vi "Get Exponent of a Number (U32).vi"(9 "Input Valid":bool=TRUE, 10 "Binary Number":u32 format="%.0b") -> (1 "Output Valid":bool, 2 "Exponent":u8, 5 "Binary Number":u32)   [LabVIEW 2011]
uses:
  <vilib>/rvi/FXPMathLib/basic elements/FxpDiscreteDelay/XNode/nifxpmath_DiscreteDelay.xnode
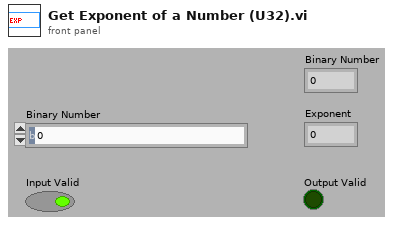
[diagram p1: front panel]
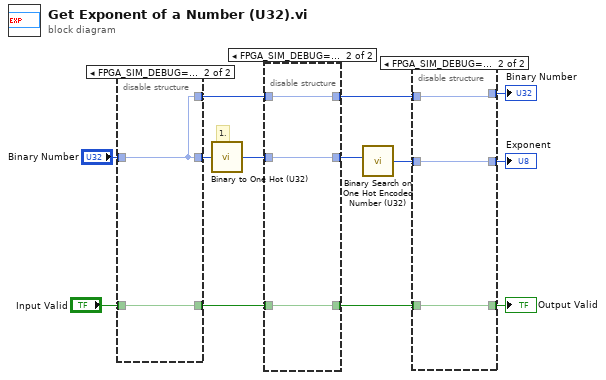
[diagram p0: block diagram]
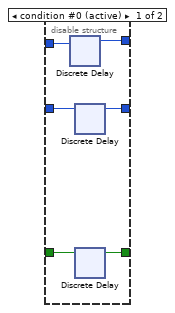
[diagram p2: hidden frame]
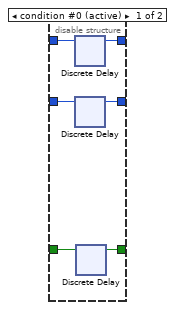
[diagram p3: hidden frame]
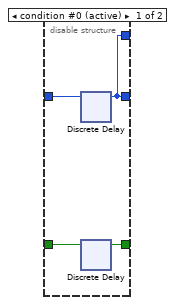
[diagram p4: hidden frame]
diagram:
  # "1."
  n1 = disable-structure shown="FPGA_SIM_DEBUG==TRUE" {
    disable-tunnel: [w14 w18] -> w13
    disable-tunnel: "Input Valid" -> [w17 w19]
    disable-tunnel: [w16 w19] -> w11
    disable-tunnel: "Binary Number" -> [w15 w18]
    disable-tunnel: [w14 w18] -> w3
    frame condition #0 (active) {
      n2 = xnode "Discrete Delay"("D"=w15) -> ("Q"=w14:u32)
      n3 = xnode "Discrete Delay"("D"=w17) -> ("Q"=w16:bool)
    }
    frame condition #1 {
    }
  }
  n4 = call <userlib>:"Binary to One Hot (U32).vi"("Binary Number"=w13) -> ("One Hot Encoded Number"=w9:u32)  [unwired: 14 in]
  n5 = disable-structure shown="FPGA_SIM_DEBUG==TRUE" {
    disable-tunnel: w11 -> [w25 w27]
    disable-tunnel: [w24 w27] -> w10
    disable-tunnel: w9 -> [w23 w28]
    disable-tunnel: [w22 w28] -> w8
    disable-tunnel: w3 -> [w21 w26]
    disable-tunnel: [w20 w26] -> w2
    frame condition #0 (active) {
      n6 = xnode "Discrete Delay"("D"=w21) -> ("Q"=w20:u32)
      n7 = xnode "Discrete Delay"("D"=w23) -> ("Q"=w22:u32)
      n8 = xnode "Discrete Delay"("D"=w25) -> ("Q"=w24:bool)
    }
    frame condition #1 {
    }
  }
  n9 = call <userlib>:"Binary Search on One Hot Encoded Number (U32).vi"("One Hot Encoded Number"=w8) -> ("Binary Number"=w6:u8)  [unwired: 14 in]
  n10 = disable-structure shown="FPGA_SIM_DEBUG==TRUE" {
    disable-tunnel: [w34 w37] -> w5
    disable-tunnel: [w33 w36] -> w4
    disable-tunnel: w10 -> [w32 w36]
    disable-tunnel: w6 -> [w31 w37]
    disable-tunnel: w2 -> [w30 w35]
    disable-tunnel: [w29 w35] -> w1
    frame condition #0 (active) {
      n11 = xnode "Discrete Delay"("D"=w30) -> ("Q"=w29:u32)
      n12 = xnode "Discrete Delay"("D"=w31) -> ("Q"=w34:u8)
      n13 = xnode "Discrete Delay"("D"=w32) -> ("Q"=w33:bool)
    }
    frame condition #1 {
    }
  }
  "Exponent" <- w5
  "Output Valid" <- w4
  "Binary Number" <- w1
